vi "DigitalInput-DAQmxReadByDevice.vi"(8 "error in":errorcluster, 9 "Num lines":i32, 10 "Original indices":i32[][](array[numeric]), 11 "Tasks by device":refnum<k21>[](array[refnum])) -> (0 "error out":errorcluster, 2 "data":bool[](array[boolean]), 3 "Tasks (dup)":refnum<k21>[](array[refnum]))   [LabVIEW 2015]
doc: "Calls DAQmx-Read, Digital 1D Bool, 1 Chan 1 Samp on an array of tasks, then recompiles their outputs into a single 1D Boolean array based on the mapping in \"Original indices\""
uses:
  <vilib>/DAQmx/read.llb/DAQmx Read (Digital 1D Bool 1Chan 1Samp).vi
  <vilib>/DAQmx/miscellaneous.llb/DAQmx Fill In Error Info.vi
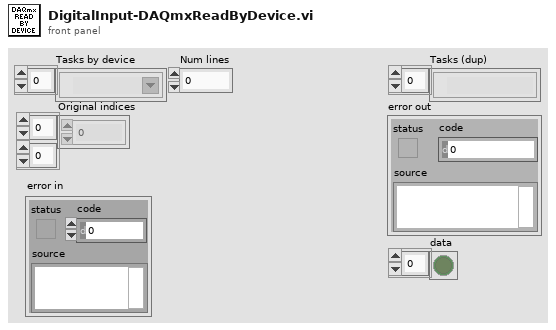
[diagram p1: front panel]
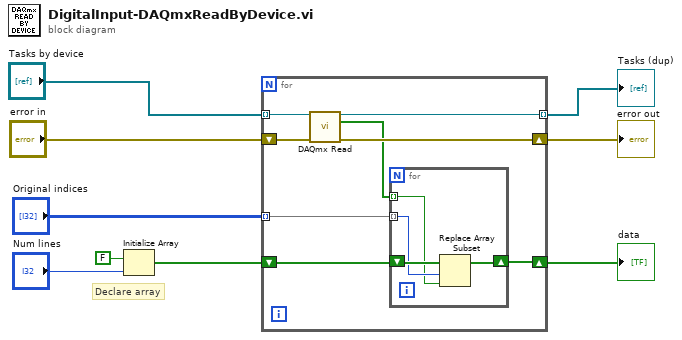
[diagram p0: block diagram]
diagram:
  # "Declare array"
  n1 = Initialize Array(FALSE, "Num lines") -> (w2:bool[])
  n2 = for {
    tunnel: "Tasks by device" -> [w16] mode=indexing
    shift-right: [w15] -> w4
    shift-left: "error in" -> [w17]
    tunnel: [w14] -> w5 mode=indexing
    tunnel: "Original indices" -> [w12] mode=indexing
    shift-right: [w10] -> w1
    shift-left: w2 -> [w11]
    n3 = call-poly <vilib>:"DAQmx Read.vi"("task/channels in"=w16, "error in"=w17) -> ("task out"=w14:refnum<k21>, "data"=w13:bool[], "error out"=w15:errorcluster)  [unwired: 11 in]
    n4 = for {
      tunnel: w13 -> [w19] mode=indexing
      tunnel: w12 -> [w20] mode=indexing
      shift-right: [w18] -> w10
      shift-left: w11 -> [w21]
      n5 = Replace Array Subset(array=w21, new element=w19, index=w20) -> (w18:bool[])
    }
  }
  "Tasks (dup)" <- w5
  "error out" <- w4
  "data" <- w1
